vi "Reboot ESC module.vi"() -> (0 "Error out":errorcluster)   [LabVIEW 2021]
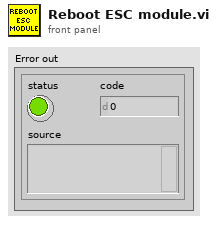
[diagram p1: front panel]
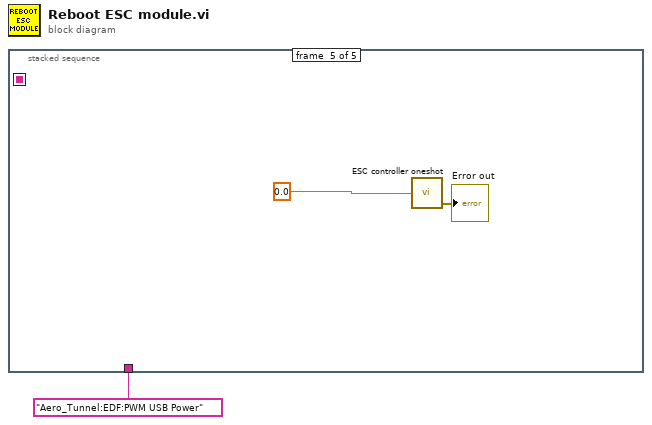
[diagram p0: block diagram]
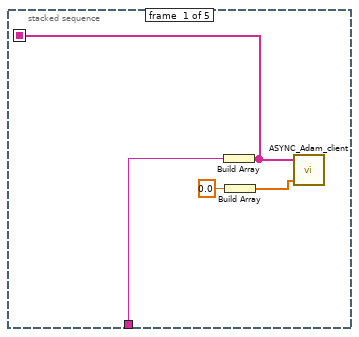
[diagram p2: hidden frame]
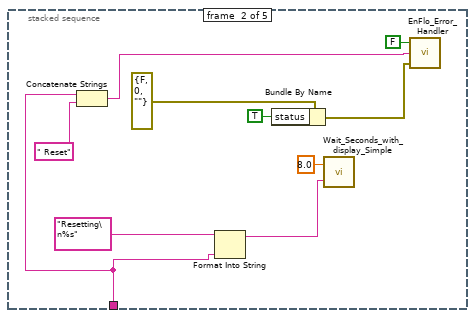
[diagram p3: hidden frame]
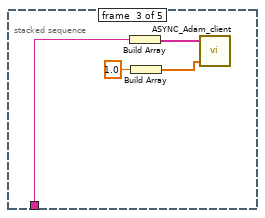
[diagram p4: hidden frame]
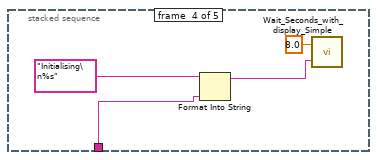
[diagram p5: hidden frame]
diagram:
  n1 = stacked-sequence {
    seq-local: [w3 _ _ _ _] -> [_ _ _ _ _]
    tunnel: "Aero_Tunnel:EDF:PWM USB Power" -> [w2 w8 w17 w22 _]
    frame #0 {
      n2 = Build Array(w2) -> (w3:string[])
      n3 = Build Array(0.0 ("element")) -> (w5:dbl[])
      n4 = call "ASYNC_Adam_client.vi"("Values"=w5, "Channel Names"=w3) -> ()  [unwired: 1 in, 2 out]
    }
    frame #1 {
      n5 = Concatenate Strings(w8, " Reset" ("string")) -> (w7:string)
      n6 = Format Into String(format string="Resetting\n%s", w8) -> (resulting string=w13:string)  [unwired: 2 in, 1 out]
      n7 = Bundle By Name(cluster=errorcluster {"status"=FALSE, "code"=0, "source"=""} ("error in (no error)"), "status"=TRUE) -> (w9:errorcluster)
      n8 = call "Wait_Seconds_with_display_Simple.vi"("Message"=w13, "Seconds to wait"=8.0) -> ()  [unwired: 1 in, 1 out]
      n9 = call "EnFlo_Error_Handler.vi"("error in (no error)"=w9, "Error Type"=w7, "Dialog Box (F)"=FALSE) -> ()  [unwired: 1 in, 2 out]
    }
    frame #2 {
      n10 = Build Array(w17) -> (w16:string[])
      n11 = Build Array(1.0 ("element")) -> (w19:dbl[])
      n12 = call "ASYNC_Adam_client.vi"("Values"=w19, "Channel Names"=w16) -> ()  [unwired: 1 in, 2 out]
    }
    frame #3 {
      n13 = Format Into String(format string="Initialising\n%s", w22) -> (resulting string=w20:string)  [unwired: 2 in, 1 out]
      n14 = call "Wait_Seconds_with_display_Simple.vi"("Message"=w20, "Seconds to wait"=8.0) -> ()  [unwired: 1 in, 1 out]
    }
    frame #4 {
      n15 = call "ESC controller oneshot.vi"("Output %"=sgl 0.0) -> ("Error out"=→"Error out":errorcluster)  [unwired: 4 in]
    }
  }
